vi "con_sub_tec_data.vi"(3 "file path":path) -> (1 "output array":dbl[](array[numeric]))   [LabVIEW 2018]
panel:
  out "line":string
  out "Iteration":i32
  out "Extracted Numbers":dbl[](array[numeric]) format="%#.6g"
  out "con sub tec output":dbl[][](array[numeric])
  out "ROIC_Temp_max":dbl
  out "ROIC_Temp_min":dbl
  out "BASE_Temp_max":dbl
  out "BASE_Temp_min":dbl
  out "ROIC_Duty_max":dbl
  out "ROIC_Duty_min":dbl
  out "RCVR_Temp_max":dbl
  out "RCVR_Temp_min":dbl
  out "No. lines":i32
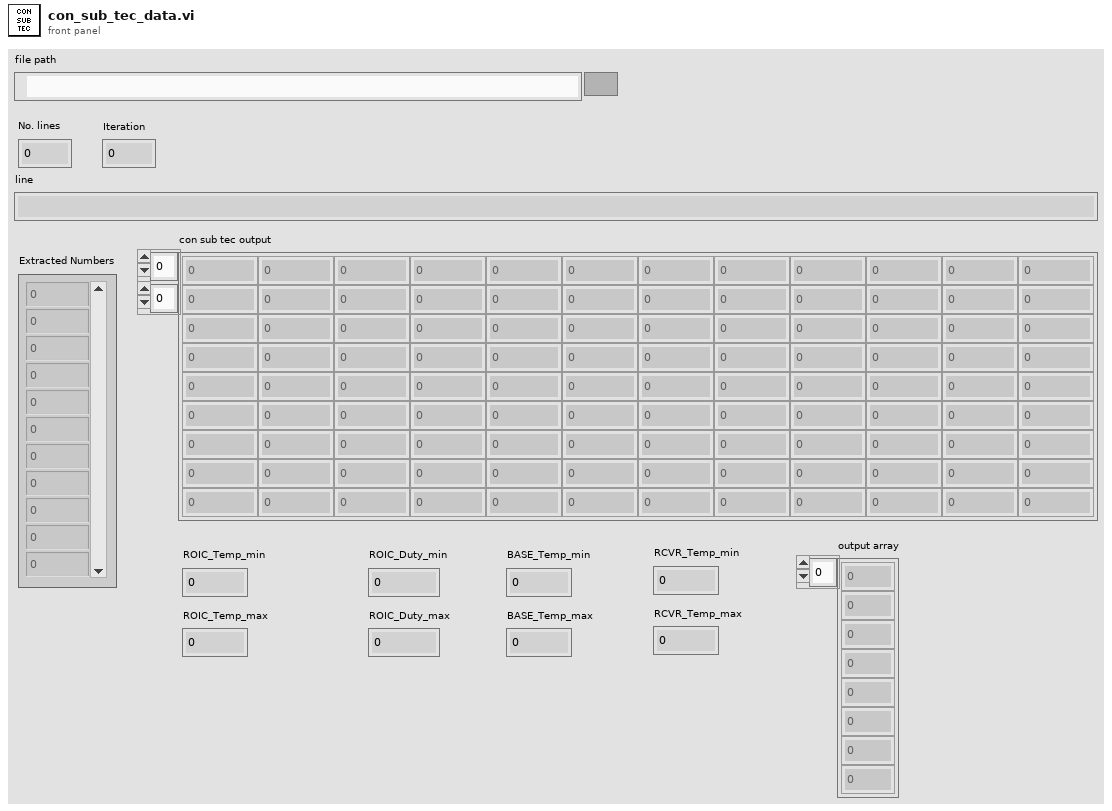
[diagram p1: front panel]
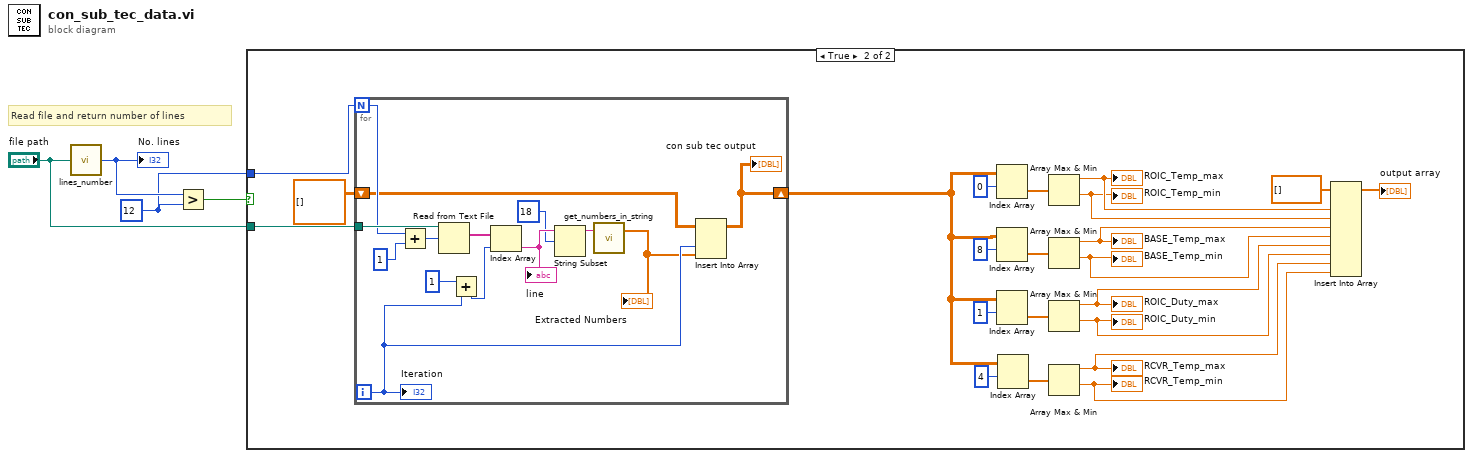
[diagram p0: block diagram]
diagram:
  w1 = 12 ("y")
  # "Read file and return number of lines"
  n1 = call "lines_number.vi"("file path"="file path") -> ("No. lines"=w3:i32)
  "No. lines" <- w3
  n2 = Greater?(x=w3, y=w1) -> (0:w4:bool)
  n3 = case shown="True" w4 {
    tunnel: "file path" -> [_ w26]
    tunnel: w1 -> [_ w25]
    frame False {
      # "If fail to get required lines execute 'hbEnable 1' again"
    }
    frame True {
      n4 = for {
        N: w25 -> [w33]
        tunnel: w26 -> [w40]
        shift-right: [w30] -> w15
        shift-left: dbl[][] [] -> [w29]
        i -> [w32]
        n5 = Add(x=w33, y=1) -> (x+y=w34:i32)
        n6 = Read from Text File(file (use dialog)=w40, count=w34) -> (text=w39:string[])  [unwired: 2 in, 3 out]
        n7 = Add(x=1, y=w32) -> (x+y=w36:i32)
        n8 = Index Array(array=w39, index=w36) -> (element=w38:string)
        "line" <- w38
        n9 = String Subset(string=w38, offset (0)=18) -> (substring=w28:string)  [unwired: 1 in]
        n10 = call "get_numbers_in_string.vi"("String"=w28) -> ("Extracted Numbers"=w31:dbl[])  [unwired: 1 in, 1 out]
        "Extracted Numbers" <- w31
        n11 = Insert Into Array(array=w29, index (col)=w32, new element=w31) -> (w30:dbl[][])  [unwired: 1 in]
        "con sub tec output" <- w30
        "Iteration" <- w32
      }
      n12 = Index Array(array=w15, index (row)=0) -> (element=w23:dbl[])  [unwired: 1 in]
      n13 = Index Array(array=w15, index (row)=8) -> (element=w21:dbl[])  [unwired: 1 in]
      n14 = Index Array(array=w15, index (row)=1) -> (element=w19:dbl[])  [unwired: 1 in]
      n15 = Index Array(array=w15, index (row)=4) -> (element=w17:dbl[])  [unwired: 1 in]
      n16 = Array Max & Min(array=w23) -> (max value=w14:dbl, min value=w13:dbl)  [unwired: 2 out]
      "ROIC_Temp_max" <- w14
      "ROIC_Temp_min" <- w13
      n17 = Array Max & Min(array=w21) -> (max value=w12:dbl, min value=w11:dbl)  [unwired: 2 out]
      "BASE_Temp_max" <- w12
      "BASE_Temp_min" <- w11
      n18 = Array Max & Min(array=w19) -> (max value=w10:dbl, min value=w7:dbl)  [unwired: 2 out]
      "ROIC_Duty_max" <- w10
      "ROIC_Duty_min" <- w7
      n19 = Array Max & Min(array=w17) -> (max value=w6:dbl, min value=w5:dbl)  [unwired: 2 out]
      "RCVR_Temp_max" <- w6
      "RCVR_Temp_min" <- w5
      n20 = Insert Into Array(array=dbl[] [], new element #1=w14, new element #2=w13, new element #3=w12, new element #4=w11, new element #5=w10, new element #6=w7, new element #7=w6, new element #8=w5) -> (→"output array":dbl[])  [unwired: 1 in]
    }
  }
